vi "svfa_Tone Estimation.vi"   [LabVIEW 2017]
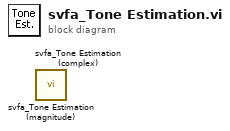
[diagram p0: block diagram]
diagram:
  n1 = call <vilib>:"svfa_Tone Estimation (magnitude).vi"() -> ()  [unwired: 11 in, 1 out]
  n2 = call <vilib>:"svfa_Tone Estimation (complex).vi"() -> ()  [unwired: 11 in, 1 out]
